vi "Squence_to_Array_SubVI.vi"(11 "Sequence":T1) -> (3 "Array":cluster{"Timing 0":dbl[]}[](array[cluster]))   [LabVIEW 2021]
uses:
  Addons/DAQ_Pulse_Gen/DAQ_Control_1.ctl
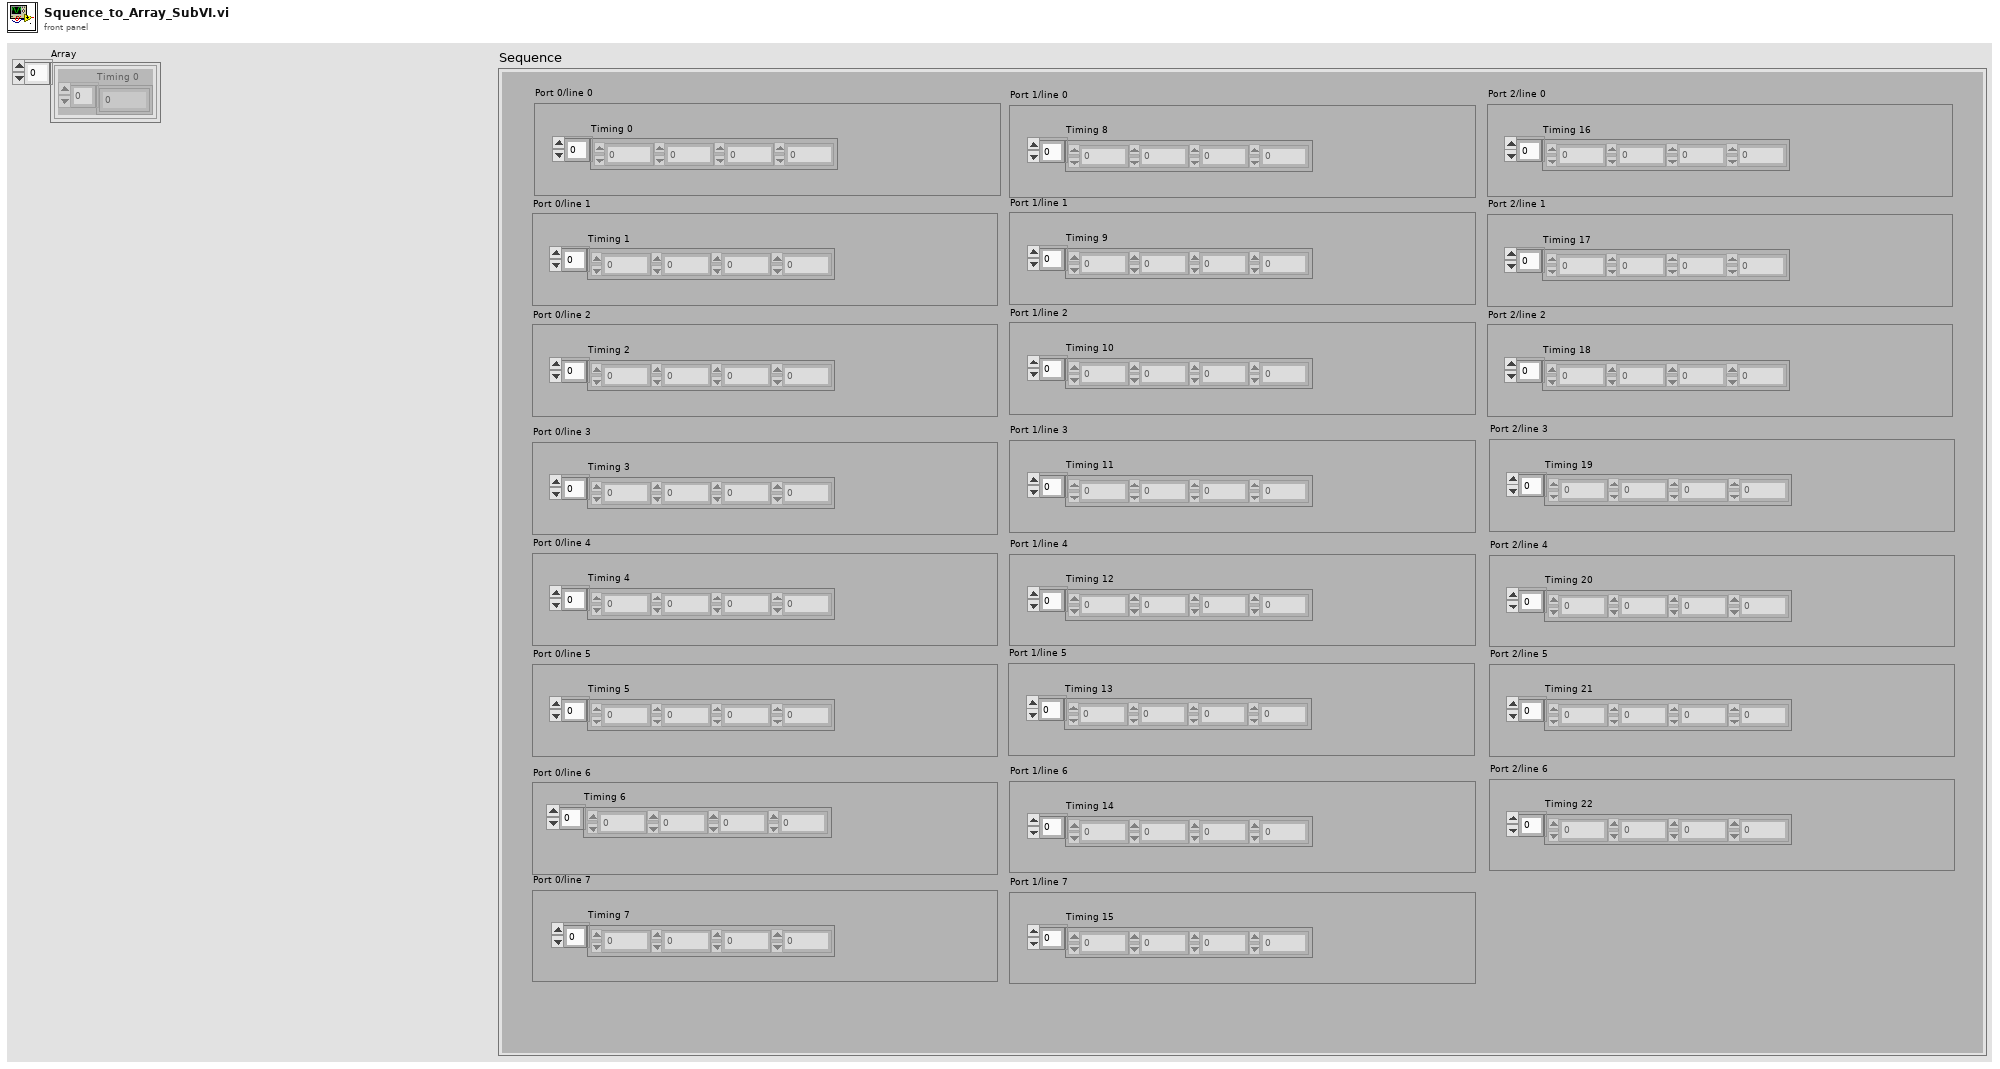
[diagram p1: front panel]
types:
  T1 = typedef "DAQ_Control_1.ctl" = cluster{"Port 2/line 6":cluster{"Timing 22":dbl[]}, "Port 2/line 5":cluster{"Timing 21":dbl[]}, "Port 2/line 4":cluster{"Timing 20":dbl[]}, "Port 2/line 3":cluster{"Timing 19":dbl[]}, "Port 2/line 2":cluster{"Timing 18":dbl[]}, "Port 2/line 1":cluster{"Timing 17":dbl[]}, "Port 2/line 0":cluster{"Timing 16":dbl[]}, "Port 1/line 7":cluster{"Timing 15":dbl[]}, "Port 1/line 6":cluster{"Timing 14":dbl[]}, "Port 1/line 5":cluster{"Timing 13":dbl[]}, "Port 1/line 4":cluster{"Timing 12":dbl[]}, "Port 1/line 3":cluster{"Timing 11":dbl[]}, "Port 1/line 2":cluster{"Timing 10":dbl[]}, "Port 1/line 1":cluster{"Timing 9":dbl[]}, "Port 1/line 0":cluster{"Timing 8":dbl[]}, "Port 0/line 7":cluster{"Timing 7\n":dbl[]}, "Port 0/line 6":cluster{"Timing 6\n":dbl[]}, "Port 0/line 5":cluster{"Timing 5\n":dbl[]}, "Port 0/line 4":cluster{"Timing 4\n":dbl[]}, "Port 0/line 3":cluster{"Timing 3\n":dbl[]}, "Port 0/line 2":cluster{"Timing 2":dbl[]}, "Port 0/line 1":cluster{"Timing 1\n":dbl[]}, "Port 0/line 0":cluster{"Timing 0":dbl[]}}
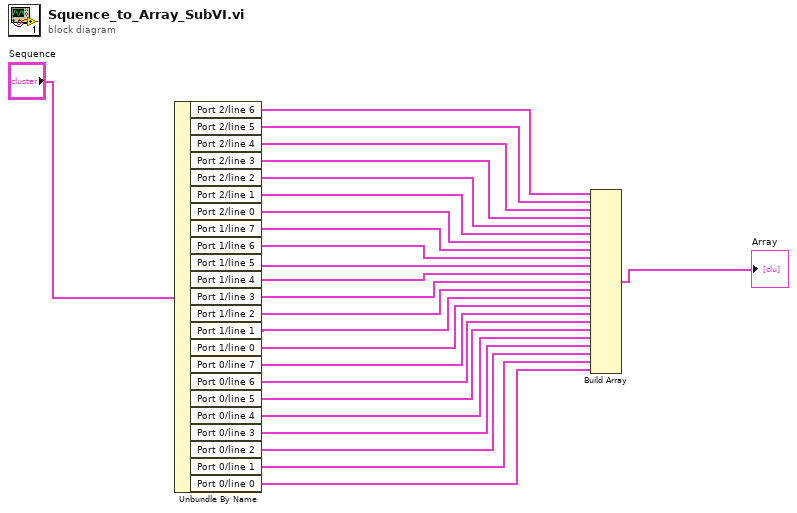
[diagram p0: block diagram]
diagram:
  n1 = Unbundle By Name("Sequence") -> ("Port 2/line 6"=w24:cluster{"Timing 22":dbl[]}, "Port 2/line 5"=w23:cluster{"Timing 21":dbl[]}, "Port 2/line 4"=w22:cluster{"Timing 20":dbl[]}, "Port 2/line 3"=w21:cluster{"Timing 19":dbl[]}, "Port 2/line 2"=w20:cluster{"Timing 18":dbl[]}, "Port 2/line 1"=w18:cluster{"Timing 17":dbl[]}, "Port 2/line 0"=w17:cluster{"Timing 16":dbl[]}, "Port 1/line 7"=w16:cluster{"Timing 15":dbl[]}, "Port 1/line 6"=w15:cluster{"Timing 14":dbl[]}, "Port 1/line 5"=w14:cluster{"Timing 13":dbl[]}, "Port 1/line 4"=w4:cluster{"Timing 12":dbl[]}, "Port 1/line 3"=w3:cluster{"Timing 11":dbl[]}, "Port 1/line 2"=w2:cluster{"Timing 10":dbl[]}, "Port 1/line 1"=w1:cluster{"Timing 9":dbl[]}, "Port 1/line 0"=w13:cluster{"Timing 8":dbl[]}, "Port 0/line 7"=w12:cluster{"Timing 7\n":dbl[]}, "Port 0/line 6"=w11:cluster{"Timing 6\n":dbl[]}, "Port 0/line 5"=w10:cluster{"Timing 5\n":dbl[]}, "Port 0/line 4"=w9:cluster{"Timing 4\n":dbl[]}, "Port 0/line 3"=w8:cluster{"Timing 3\n":dbl[]}, "Port 0/line 2"=w7:cluster{"Timing 2":dbl[]}, "Port 0/line 1"=w6:cluster{"Timing 1\n":dbl[]}, "Port 0/line 0"=w5:cluster{"Timing 0":dbl[]})
  n2 = Build Array(w24, w23, w22, w21, w20, w18, w17, w16, w15, w14, w4, w3, w2, w1, w13, w12, w11, w10, w9, w8, w7, w6, w5) -> (→"Array":cluster{"Timing 0":dbl[]}[])
